vi "LL_GET Service.vi"(8 "error in (no error)":errorcluster) -> (0 "error out":errorcluster, 1 "Call Result":T4, 3 "ListAllMyBucketsResult":T1)   [LabVIEW 2011, in "LV Interface for Amazon S3.lvlib"]
doc: "This implementation of the GET operation returns a list of all buckets owned by the authenticated sender of the request. Use this VI instead of the <B>List Buckets.vi</B> if you need more iformation than that returned by that VI."
uses:
  LV Interface for Amazon S3.lvlib
  Typedefs/AMZ_S3_Call Results.ctl
  Typedefs/AMZ_S3_API_ListAllMyBucketsResult.ctl
  Typedefs/AMZ_S3_API_Owner.ctl
  Typedefs/AMZ_S3_API_Bucket.ctl
  <vilib>/httpClient/LabVIEWHTTPClient.lvlib
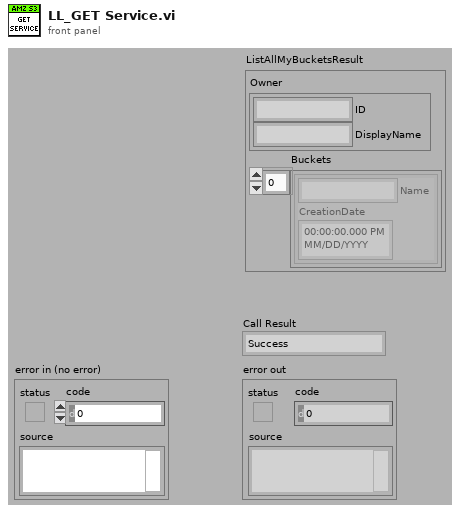
[diagram p1: front panel]
types:
  T1 = typedef "LV Interface for Amazon S3.lvlib/AMZ_S3_API_ListAllMyBucketsResult.ctl" = cluster{"Owner":T2, "Buckets":T3[]}
  T2 = typedef "LV Interface for Amazon S3.lvlib/AMZ_S3_API_Owner.ctl" = cluster{"ID":string, "DisplayName":string}
  T3 = typedef "LV Interface for Amazon S3.lvlib/AMZ_S3_API_Bucket.ctl" = cluster{"Name":string, "CreationDate":timestamp}
  T4 = typedef "LV Interface for Amazon S3.lvlib/AMZ_S3_Call Results.ctl" = enum16{"Success", "UndefinedError", "AccessDenied", "AccountProblem", "AmbiguousGrantByEmailAddress", "BadDigest", "BucketAlreadyExists", "BucketAlreadyOwnedByYou", "BucketNotEmpty", "CredentialsNotSupported", "CrossLocationLoggingProhibited", "EntityTooSmall", "EntityTooLarge", "ExpiredToken", "IllegalVersioningConfigurationException", "IncompleteBody", "IncorrectNumberOfFilesInPostRequest", "InlineDataTooLarge", "InternalError", "InvalidAccessKeyId", "InvalidAddressingHeader", "InvalidArgument", "InvalidBucketName", "InvalidDigest", "InvalidLocationConstraint", "InvalidPart", "InvalidPartOrder", "InvalidPayer", "InvalidPolicyDocument", "InvalidRange", "InvalidSecurity", "InvalidSOAPRequest", "InvalidStorageClass", "InvalidTargetBucketForLogging", "InvalidToken", "InvalidURI", "KeyTooLong", "MalformedACLError", "MalformedPOSTRequest", "MalformedXML", "MaxMessageLengthExceeded", "MaxPostPreDataLengthExceededError", "MetadataTooLarge", "MethodNotAllowed", "MissingAttachment", "MissingContentLength", "MissingRequestBodyError", "MissingSecurityElement", "MissingSecurityHeader", "NoLoggingStatusForKey", "NoSuchBucket", "NoSuchKey", "NoSuchUpload", "NoSuchVersion", "NotImplemented", "NotSignedUp", "OperationAborted", "PermanentRedirect", "PreconditionFailed", "Redirect", "RequestIsNotMultiPartContent", "RequestTimeout", "RequestTimeTooSkewed", "RequestTorrentOfBucketError", "SignatureDoesNotMatch", "SlowDown", "TemporaryRedirect", "TokenRefreshRequired", "TooManyBuckets", "UnexpectedContent", "UnresolvableGrantByEmailAddress", "UserKeyMustBeSpecified", "LabVIEWError"}
  T5 = typedef "LabVIEWHTTPClient.lvlib/ClientHandle.ctl" = refnum<k1>
  T6 = cluster{"Value":string, "Time Stamp":timestamp}[]
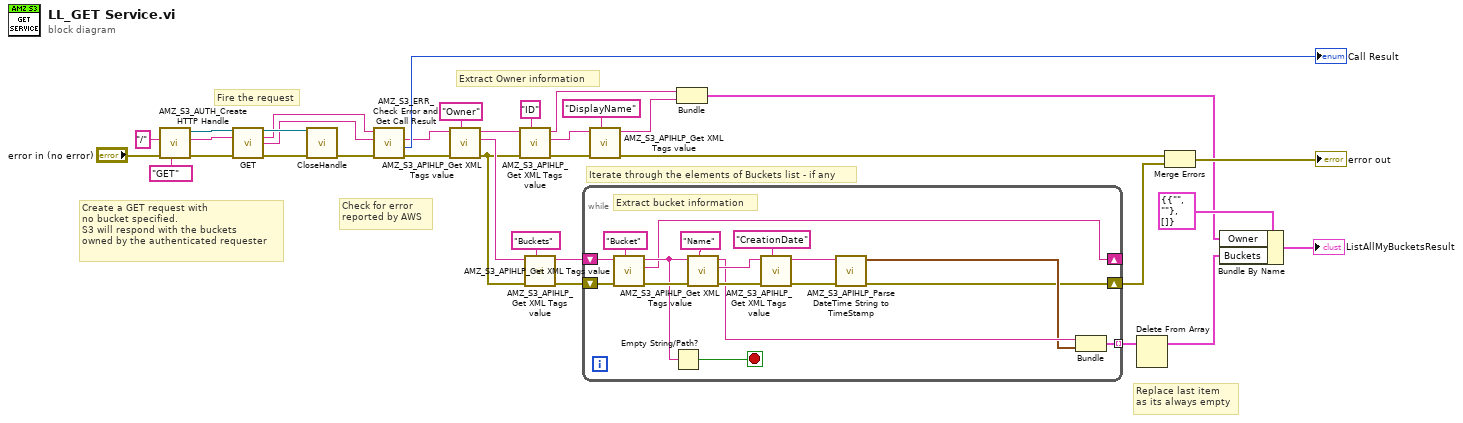
[diagram p0: block diagram]
diagram:
  # "Check for error\nreported by AWS"
  # "Fire the request"
  # "Iterate through the elements of Buckets list - if any"
  # "Extract Owner information"
  # "Replace last item\nas its always empty"
  # "Create a GET request with\nno bucket specified.\nS3 will respond with the buckets\nowned by the authenticated requester"
  n1 = call "AMZ_S3_AUTH_Create HTTP Handle.vi"("HTTP-Verb"="GET", "error in (no error)"="error in (no error)", "Path and query string"="/") -> ("error out"=w33:errorcluster, "URL"=w32:string, "client handle out"=w31:T5)  [unwired: 6 in]
  n2 = call <vilib>:"GET.vi"("client handle"=w31, "url"=w32, "error in (no error)"=w33) -> ("client handle out"=w29:T5, "headers"=w27:string, "body"=w26:string, "error out"=w30:errorcluster)  [unwired: 9 in]
  n3 = call <vilib>:"CloseHandle.vi"("client handle"=w29, "error in (no error)"=w30) -> ("error out"=w28:errorcluster)  [unwired: 13 in]
  n4 = call "AMZ_S3_ERR_Check Error and Get Call Result.vi"("error in (no error)"=w28, "Response body"=w26, "Response header"=w27) -> ("error out"=w24:errorcluster, "Call Result"=→"Call Result":T4, "Response body dup"=w23:string)  [unwired: 4 in, 2 out]
  n5 = call "AMZ_S3_APIHLP_Get XML Tags value.vi"("Tag name"="Owner", "error in (no error)"=w24, "XML String in"=w23) -> ("error out"=w13:errorcluster, "Remaining string"=w14:string, "Value"=w21:string)  [unwired: 6 in]
  n6 = call "AMZ_S3_APIHLP_Get XML Tags value.vi"("Tag name"="ID", "error in (no error)"=w13, "XML String in"=w21) -> ("error out"=w19:errorcluster, "Remaining string"=w18:string, "Value"=w15:string)  [unwired: 6 in]
  n7 = call "AMZ_S3_APIHLP_Get XML Tags value.vi"("Tag name"="Buckets", "error in (no error)"=w13, "XML String in"=w14) -> ("error out"=w11:errorcluster, "Value"=w10:string)  [unwired: 6 in, 1 out]
  n8 = while {
    shift-right: [w46] -> _
    shift-left: w10 -> [w51]
    tunnel: [w40] -> w9 mode=indexing
    shift-right: [w36] -> w7
    shift-left: w11 -> [w52]
    stop <- w50 stop-if-true
    # "Extract bucket information"
    n9 = call "AMZ_S3_APIHLP_Get XML Tags value.vi"("Tag name"="Bucket", "error in (no error)"=w52, "XML String in"=w51) -> ("error out"=w48:errorcluster, "Remaining string"=w46:string, "Value"=w47:string)  [unwired: 6 in]
    n10 = Empty String/Path?(string/path=w47) -> (empty?=w50:bool)
    n11 = call "AMZ_S3_APIHLP_Get XML Tags value.vi"("Tag name"="Name", "error in (no error)"=w48, "XML String in"=w47) -> ("error out"=w44:errorcluster, "Remaining string"=w43:string, "Value"=w41:string)  [unwired: 6 in]
    n12 = call "AMZ_S3_APIHLP_Get XML Tags value.vi"("Tag name"="CreationDate", "error in (no error)"=w44, "XML String in"=w43) -> ("error out"=w39:errorcluster, "Value"=w38:string)  [unwired: 6 in, 1 out]
    n13 = call "AMZ_S3_APIHLP_Parse DateTime String to TimeStamp.vi"("error in (no error)"=w39, "DateTime String"=w38) -> ("error out"=w36:errorcluster, "Time Stamp"=w37:timestamp)  [unwired: 8 in]
    n14 = Bundle("Value"=w41, "Time Stamp"=w37) -> (w40:cluster{"Value":string, "Time Stamp":timestamp})  [unwired: 1 in]
  }
  n15 = call "AMZ_S3_APIHLP_Get XML Tags value.vi"("Tag name"="DisplayName", "error in (no error)"=w19, "XML String in"=w18) -> ("error out"=w8:errorcluster, "Value"=w16:string)  [unwired: 6 in, 1 out]
  n16 = Bundle("Value"=w15, "Value"=w16) -> (w2:cluster{"Value":string, "Value":string})  [unwired: 1 in]
  n17 = Delete From Array(array=w9) -> (array with subset deleted=w3:T6)  [unwired: 2 in, 1 out]
  n18 = Merge Errors(w8, w7) -> (→"error out":errorcluster)
  n19 = Bundle By Name(cluster=T1 {"Owner"={"ID"="", "DisplayName"=""}, "Buckets"=[]} ("ListAllMyBucketsResult"), "Owner"=w2, "Buckets"=w3) -> (→"ListAllMyBucketsResult":T1)
